vi "Read Log Files Directory.vi"(8 "error in (no error)":errorcluster, 11 "Config Manager Class in":refnum<class "Config Manager Class.lvclass">) -> (0 "error out":errorcluster, 2 "Log Files Directory":path, 3 "Config Manager Class out":refnum<class "Config Manager Class.lvclass">)   [LabVIEW 2017, in "Config Manager Class.lvclass"]
uses:
  Config Manager Class.lvclass
  Config Manager Class.lvclass/Config Manager Class.ctl
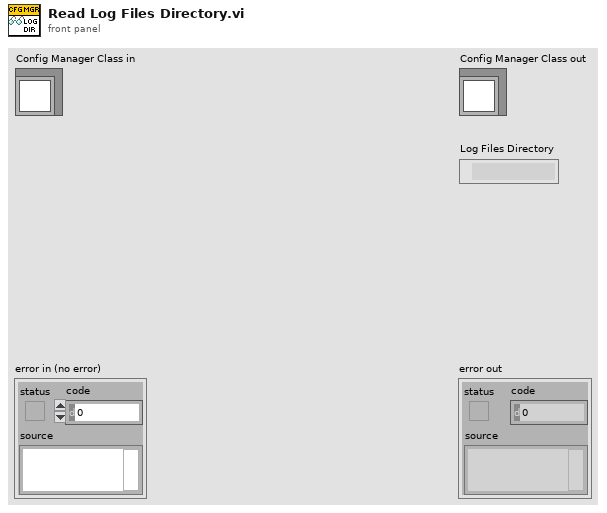
[diagram p1: front panel]
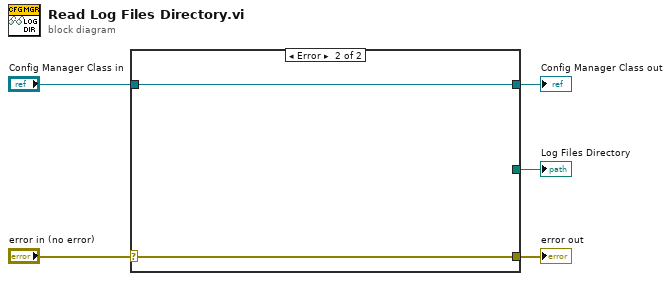
[diagram p0: block diagram]
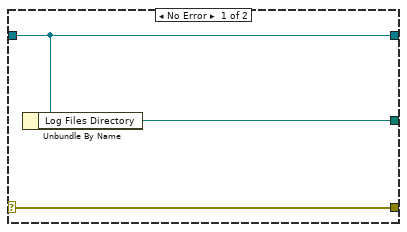
[diagram p2: hidden frame]
diagram:
  n1 = case shown="Error" "error in (no error)" {
    selector: "error in (no error)" -> [w8 w9]
    tunnel: [w8 w9] -> w4
    tunnel: [w7 w10] -> w2
    tunnel: "Config Manager Class in" -> [w7 w10]
    tunnel: [w6 _] -> w1
    frame No Error {
      n2 = Unbundle By Name(w7) -> ("Log Files Directory"=w6:path)
    }
    frame Error {
    }
  }
  "error out" <- w4
  "Config Manager Class out" <- w2
  "Log Files Directory" <- w1
